vi "Intake Intake.vi"(1 "Intake Info In":T2) -> (0 "Intake Info Out":T2)   [LabVIEW 2013]
uses:
  <vilib>/Rock Robotics/WPI/Solenoid/WPI_SolenoidValue.ctl
panel:
  # "True = Out\nFalse = In"
  # "True = Out\nFalse = In"
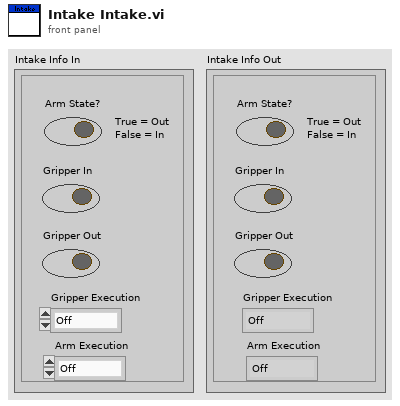
[diagram p1: front panel]
types:
  T1 = typedef "WPI_SolenoidValue.ctl" = enum16{"Off", "On", "Forward", "Reverse"}
  T2 = cluster{"Arm State?":bool, "Gripper In":bool, "Gripper Out":bool, "Gripper Execution ":T1, "Arm Execution ":T1}
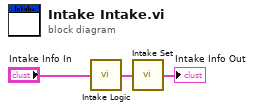
[diagram p0: block diagram]
diagram:
  n1 = call "Intake Logic.vi"("Intake Info In"="Intake Info In") -> ("Intake Info Out"=w2:T2)
  n2 = call "Intake Set.vi"("Intake Info In"=w2) -> ("Intake Info Out"=→"Intake Info Out":T2)
